vi "Constant.vi"(8 "error in":errorcluster, 11 "reference":refnum<vi>) -> (0 "error out":errorcluster, 3 "constant out":refnum<class "Constant.lvclass">)   [LabVIEW 2014, in "Raspberry Pi Compatible Compiler for LabVIEW.lvlib" / "Constant.lvclass"]
uses:
  Constant.lvclass
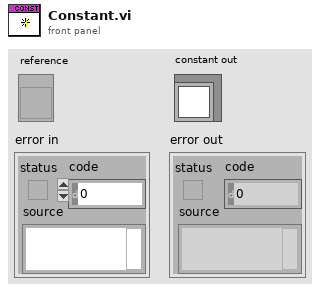
[diagram p1: front panel]
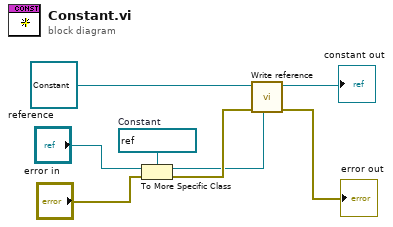
[diagram p0: block diagram]
diagram:
  w8 = refnum<vi> refnum  # Constant
  n1 = To More Specific Class(target class=w8, reference="reference", error in="error in") -> (specific class reference=w2:refnum<vi>, error out=w3:errorcluster)
  n2 = call-dynamic "Write reference.vi"("reference"=w2, "error in"=w3, "GObject in"=refnum<class "Constant.lvclass"> refnum ("constant out 2")) -> ("error out"=→"error out":errorcluster, "GObject out"=→"constant out":refnum<class "Constant.lvclass">)  [unwired: 5 in]
